vi "Calc_Force_Moment_Balance.vi"(8 "Center State at T":T2, 9 "Ini_Anchor_Posi":dbl[][](array[numeric]), 11 "On_Particle State":T1(array[cluster])) -> (0 "New Center State at T":T2, 1 "Ini_Anchor_Posi":dbl[][](array[numeric]), 3 "On_Particle State":T1(array[cluster]))   [LabVIEW 2020]
panel:
  out "SummedMoment":dbl
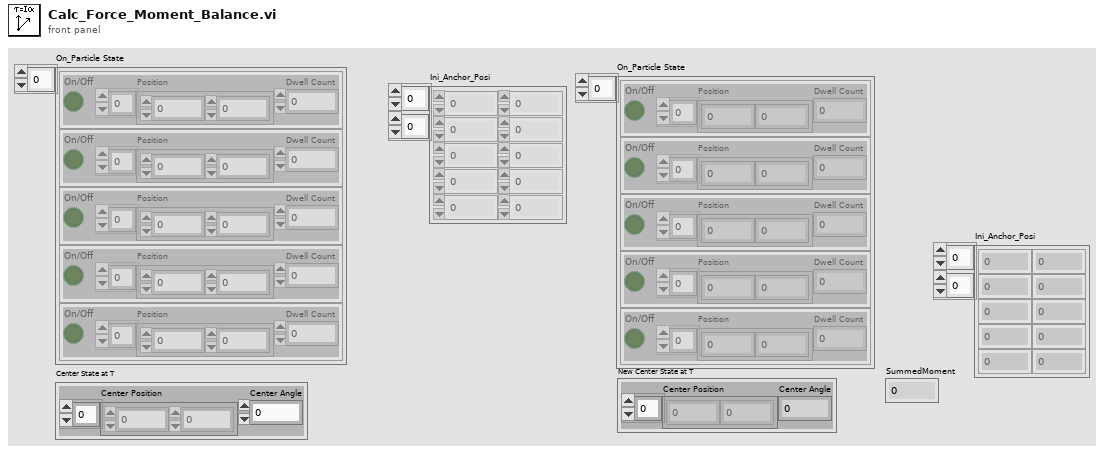
[diagram p1: front panel]
types:
  T1 = cluster{"On/Off":bool, "Position":dbl[], "Dwell Count":i32}[]
  T2 = cluster{"Center Position":dbl[], "Center Angle":dbl}
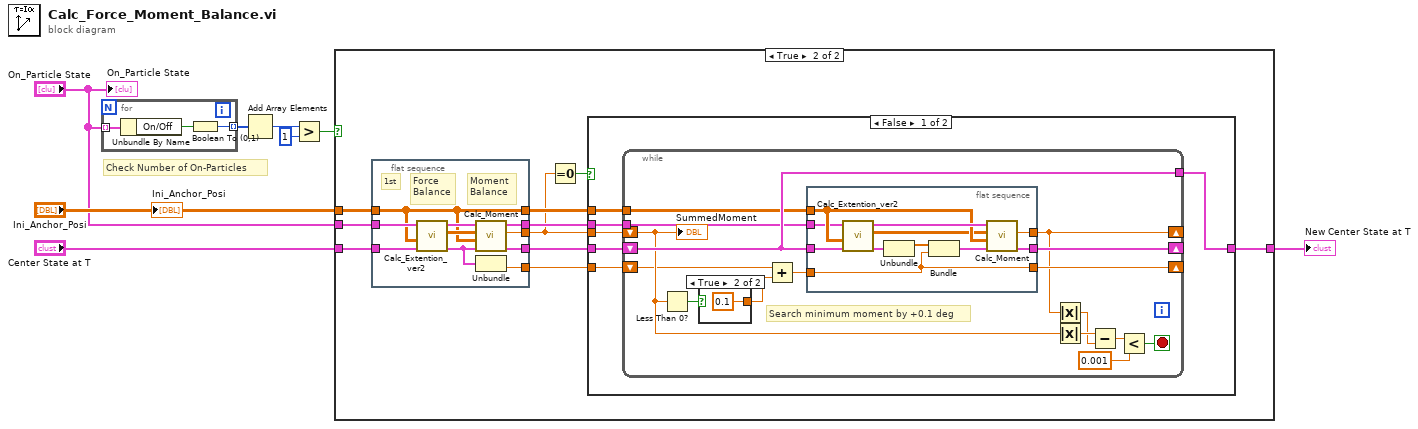
[diagram p0: block diagram]
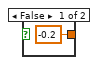
[diagram p3: hidden frame]
diagram:
  # "Check Number of On-Particles"
  n1 = for {
    tunnel: "On_Particle State" -> [w11] mode=indexing
    tunnel: [w9] -> w7 mode=indexing
    n2 = Unbundle By Name(w11) -> ("On/Off"=w10:bool)
    n3 = Boolean To (0,1)(Boolean=w10) -> (0, 1=w9:i16)
  }
  n4 = Add Array Elements(numeric array=w7) -> (sum=w1:i16)
  n5 = Greater?(x=w1, y=i16 1) -> (0:w5:bool)
  n6 = case shown="TRUE" w5 {
    tunnel: "Center State at T" -> [w12 w22]
    tunnel: "Ini_Anchor_Posi" -> [_ w20]
    tunnel: [w12 w13] -> w2
    tunnel: "On_Particle State" -> [_ w14]
    frame False {
    }
    frame True {
      n7 = flat-sequence {
        tunnel: w22 -> [w66]
        tunnel: w14 -> [w68]
        tunnel: w20 -> [w59]
        tunnel: [w65] -> w21
        tunnel: [w67] -> w19
        tunnel: [w62] -> w15
        tunnel: [w61] -> w18
        tunnel: [w59] -> w17
        frame #0 {
          # "Moment\nBalance"
          # "Force\nBalance"
          # "1st"
          n8 = call "Calc_Extention_ver2.vi"("Center State at T"=w66, "Initial Anchor Position"=w59, "On_Particle State"=w68) -> ("New Center State at T"=w60:T2, "Extension"=w64:dbl[][], "On_Particle State"=w63:T1)  [unwired: 6 in]
          n9 = call "Calc_Moment.vi"("Center State at T"=w60, "Initial Anchor Position"=w59, "Extention"=w64, "On_Particle State"=w63) -> ("Center State at T 2"=w65:T2, "SummedMoment"=w62:dbl, "On_Particle State"=w61:T1)  [unwired: 5 in]
          n10 = Unbundle(w60) -> ("Center Angle"=w67:dbl)  [unwired: 1 out]
        }
      }
      n11 = Equal To 0?(x=w15) -> (x = 0?=w16:bool)
      n12 = case shown="FALSE" w16 {
        tunnel: w21 -> [w28 w58]
        tunnel: w19 -> [w27 _]
        tunnel: [w26 w58] -> w13
        tunnel: w15 -> [w25 _]
        tunnel: w18 -> [w24 _]
        tunnel: w17 -> [w23 _]
        frame False {
          n13 = while {
            shift-right: [w29] -> _
            shift-left: w25 -> [w39]
            shift-right: [w40] -> _
            shift-left: w28 -> [w41]
            shift-right: [w33] -> _
            shift-left: w27 -> [w35]
            tunnel: [w41] -> w26
            tunnel: w24 -> [w38]
            tunnel: w23 -> [w36]
            stop <- w31 stop-if-true
            # "Search minimum moment by +0.1 deg"
            n14 = Less Than 0?(x=w39) -> (x < 0?=w43:bool)
            n15 = case shown="TRUE" w43 {
              tunnel: [-0.2 ("y") 0.1 ("y")] -> w34
              frame False {
              }
              frame True {
              }
            }
            n16 = Add(x=w35, y=w34) -> (x+y=w42:dbl)
            n17 = flat-sequence {
              tunnel: w36 -> [w55]
              tunnel: w41 -> [w56]
              tunnel: w42 -> [w47]
              tunnel: [w51] -> w40
              tunnel: w38 -> [w50]
              tunnel: [w49] -> w29
              tunnel: [w47] -> w33
              frame #0 {
                n18 = call "Calc_Extention_ver2.vi"("Center State at T"=w56, "Initial Anchor Position"=w55, "On_Particle State"=w50) -> ("New Center State at T"=w53:T2, "Extension"=w48:dbl[][], "On_Particle State"=w57:T1)  [unwired: 6 in]
                n19 = Unbundle(w53) -> ("Center Position"=w52:dbl[])  [unwired: 1 out]
                n20 = Bundle("Center Position"=w52, w47) -> (w54:cluster{"Center Position":dbl[], dbl})  [unwired: 1 in]
                n21 = call "Calc_Moment.vi"("Center State at T"=w54, "Initial Anchor Position"=w55, "Extention"=w48, "On_Particle State"=w57) -> ("Center State at T 2"=w51:T2, "SummedMoment"=w49:dbl)  [unwired: 5 in, 1 out]
              }
            }
            n22 = Absolute Value(x=w29) -> (abs(x)=w37:dbl)
            n23 = Absolute Value(x=w39) -> (abs(x)=w44:dbl)
            n24 = Subtract(x=w44, y=w37) -> (x-y=w32:dbl)
            n25 = Less?(x=w32, y=0.001) -> (x < y?=w31:bool)
            "SummedMoment" <- w39
          }
        }
        frame True {
        }
      }
    }
  }
  "New Center State at T" <- w2
  "On_Particle State" <- "On_Particle State"
  "Ini_Anchor_Posi" <- "Ini_Anchor_Posi"
